vi "DHTxx Test Create.vi"() -> ()   [LabVIEW 2014, in "ESP8266 WiFi Wrapper.lvlib"]
uses:
  ESP8266 WiFi Wrapper.lvlib
panel:
  out "Error Out":errorcluster
  in  "Error In":errorcluster
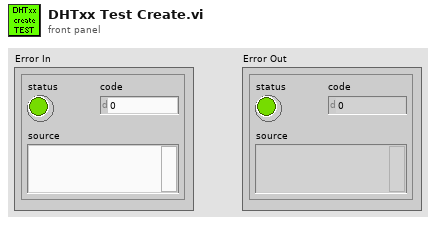
[diagram p1: front panel]
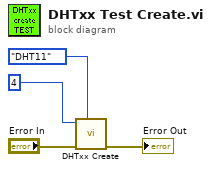
[diagram p0: block diagram]
diagram:
  n1 = call "DHTxx Create.vi"("DHT Type"=enum16{"DHT11", "DHT21", "DHT22"}."DHT11", "Error In"="Error In", "DHT pin"=u8 4) -> ("Error Out"=→"Error Out":errorcluster)  [unwired: 8 in]
